vi "Commutator_send_CMD.vi"(2 "CMD":string, 3 "VISA in":T1) -> (0 "Response":string, 1 "VISA out":T1)   [LabVIEW 2017]
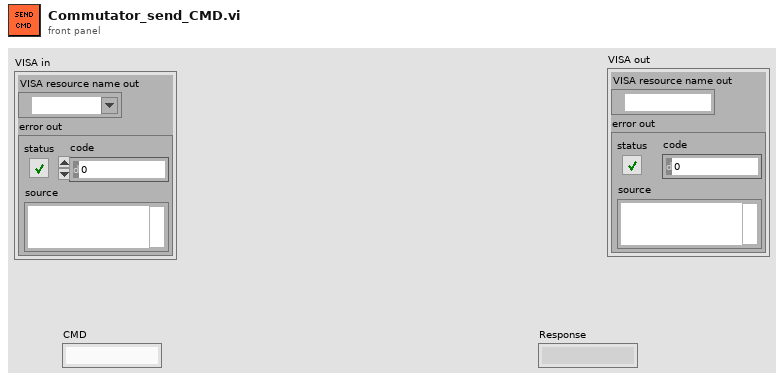
[diagram p1: front panel]
types:
  T1 = cluster{"VISA resource name out":refnum<visa-resource-name>, "error out":errorcluster}
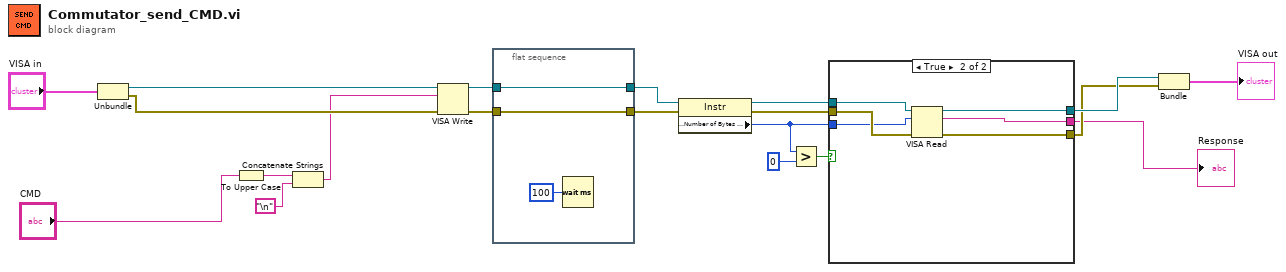
[diagram p0: block diagram]
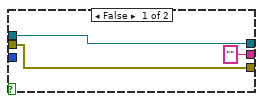
[diagram p2: hidden frame]
diagram:
  n1 = Unbundle("VISA in") -> ("VISA resource name out"=w19:refnum<visa-resource-name>, "error out"=w18:errorcluster)
  n2 = To Upper Case(1:"CMD") -> (0:w2:string)
  n3 = Concatenate Strings(w2, "\n") -> (w3:string)
  n4 = VISA Write(VISA resource name=w19, write buffer=w3, error in (no error)=w18) -> (VISA resource name out=w17:refnum<visa-resource-name>, error out=w16:errorcluster)  [unwired: 1 out]
  n5 = flat-sequence {
    tunnel: w17 -> [w22]
    tunnel: w16 -> [w21]
    tunnel: [w22] -> w15
    tunnel: [w21] -> w14
    frame #0 {
      n6 = Wait (ms)(milliseconds to wait=u32 100) -> ()  [unwired: 1 out]
    }
  }
  n7 = property class="Instr"(reference=w15, error in=w14) -> (reference out=w11:refnum<visa-resource-name>, error out=w10:errorcluster, "Serial Settings:Number of Bytes at Serial Port"=w9:u32)
  n8 = Greater?(x=w9, y=u32 0) -> (0:w13:bool)
  n9 = case shown="True" w13 {
    tunnel: w11 -> [w26 w32]
    tunnel: w10 -> [w25 w31]
    tunnel: w9 -> [_ w30]
    tunnel: [w25 w29] -> w7
    tunnel: [w26 w28] -> w8
    tunnel: ["" ("read buffer") w27] -> w5
    frame False {
    }
    frame True {
      n10 = VISA Read(VISA resource name=w32, byte count=w30, error in (no error)=w31) -> (VISA resource name out=w28:refnum<visa-resource-name>, read buffer=w27:string, error out=w29:errorcluster)  [unwired: 1 out]
    }
  }
  "Response" <- w5
  n11 = Bundle("VISA resource name out"=w8, "error out"=w7) -> (→"VISA out":T1)  [unwired: 1 in]
